vi "Create_Lineshape_P.vi"(4 "Saturation\nPolarization":dbl, 6 "Lineshape P":dbl, 7 "Microwave on":bool, 9 "Microwave Power":dbl, 10 "Relaxation Parameter":dbl, 11 "Positive Polarization\n(Flips Signal)":bool) -> (3 "Lineshape P new":dbl)   [LabVIEW 2018]
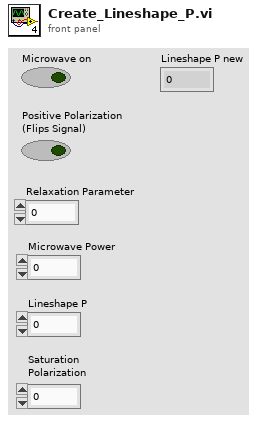
[diagram p1: front panel]
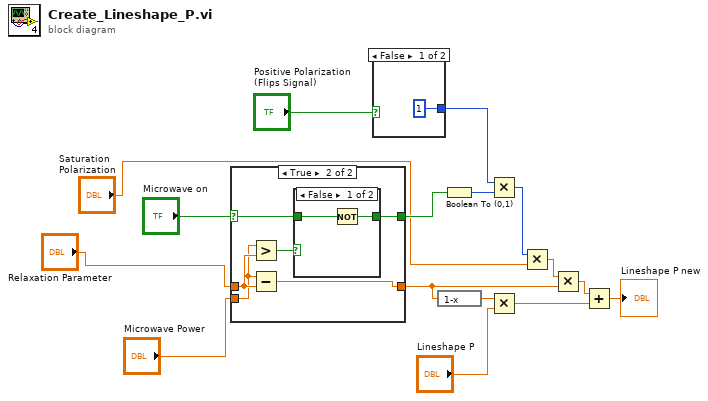
[diagram p0: block diagram]
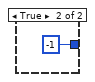
[diagram p4: hidden frame]
diagram:
  n1 = case shown="True" "Microwave on" {
    selector: "Microwave on" -> [w17 w23]
    tunnel: [w18 w19] -> w15
    tunnel: "Relaxation Parameter" -> [w18 w21]
    tunnel: [w17 w22] -> w16
    tunnel: "Microwave Power" -> [_ w20]
    frame False {
    }
    frame True {
      n2 = Greater?(x=w20, y=w21) -> (0:w24:bool)
      n3 = Subtract(x=w20, y=w21) -> (x-y=w19:dbl)
      n4 = case shown="False" w24 {
        tunnel: [w25 w27] -> w22
        tunnel: w23 -> [w26 w27]
        frame False {
          n5 = Not(x=w26) -> (.not. x?=w25:bool)
        }
        frame True {
        }
      }
    }
  }
  n6 = case shown="False" "Positive Polarization\n(Flips Signal)" {
    tunnel: [1 -1] -> w13
    frame False {
    }
    frame True {
    }
  }
  n7 = expression code="1-x"(w15) -> (w6:dbl)
  n8 = Boolean To (0,1)(Boolean=w16) -> (0, 1=w7:i16)
  n9 = Multiply(x=w13, y=w7) -> (x*y=w12:i32)
  n10 = Multiply(x=w6, y="Lineshape P") -> (x*y=w4:dbl)
  n11 = Multiply(x=w12, y="Saturation\nPolarization") -> (x*y=w10:dbl)
  n12 = Multiply(x=w10, y=w15) -> (x*y=w5:dbl)
  n13 = Add(x=w5, y=w4) -> (x+y=→"Lineshape P new":dbl)
